vi "2020_day11.vi"() -> ()   [LabVIEW 2021]
uses:
  <userlib>/_OpenG.lib/array/array.llb/Search 1D Array (String)__ogtk.vi
panel:
  out "Task 1 (# od Occupied Seats)":i32
  out "Array 2":string[][](array[string])
  out "Array":string[][](array[string])
  in  "Switch":bool caption="Ex. Data  vs.  User Data"
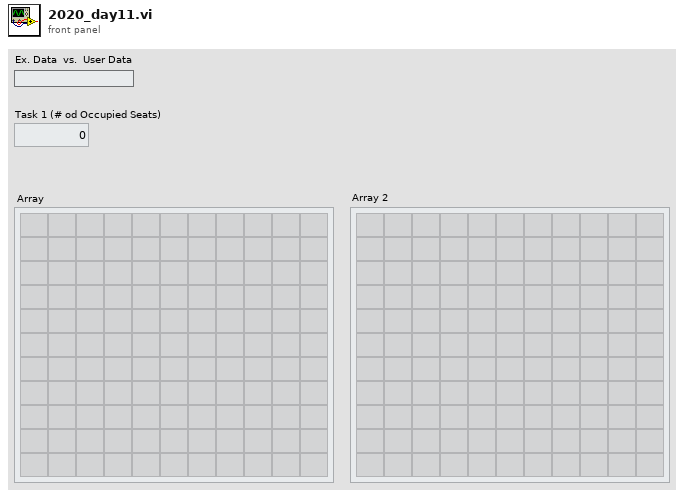
[diagram p1: front panel]
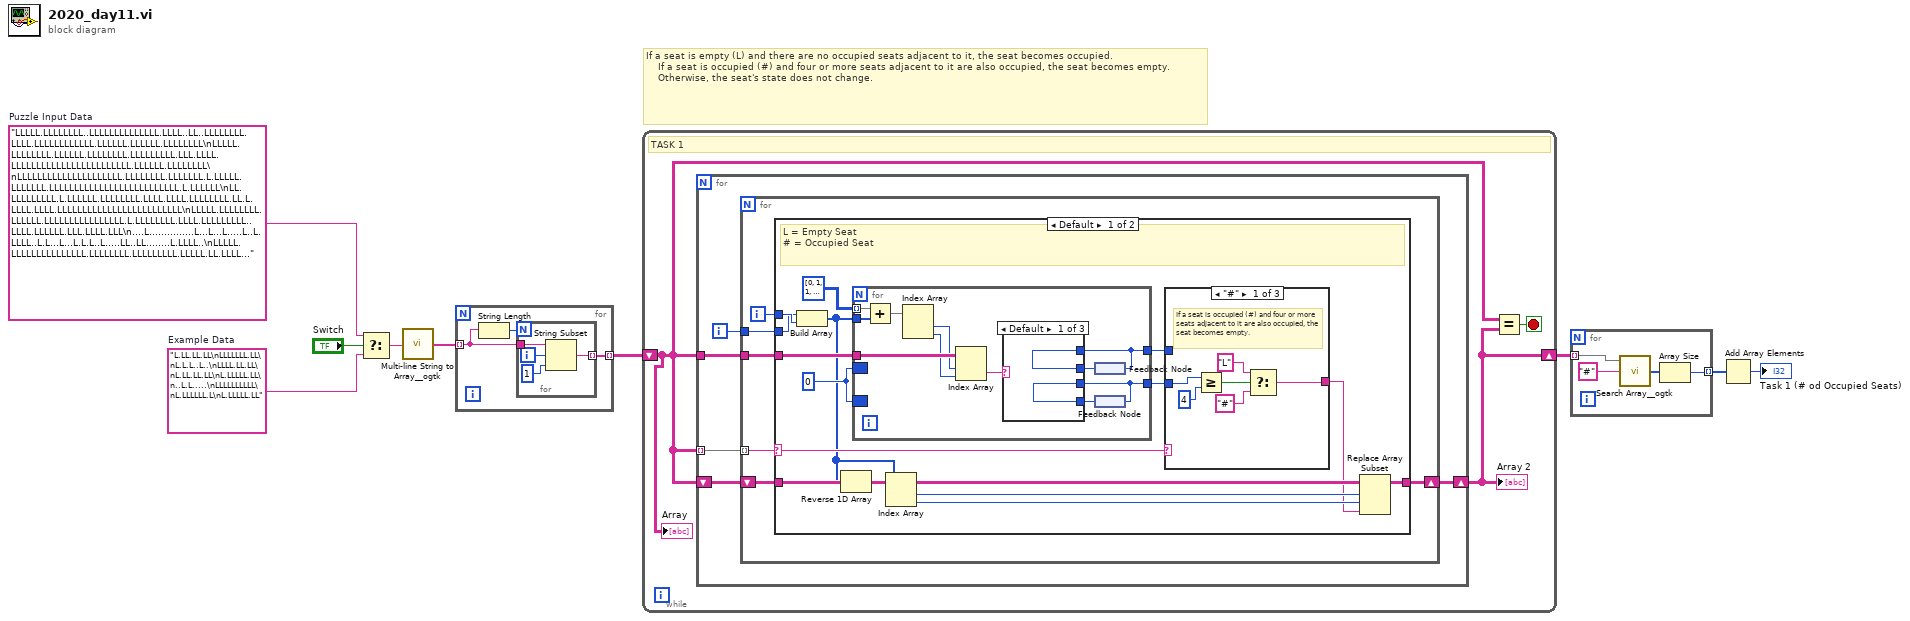
[diagram p0: block diagram]
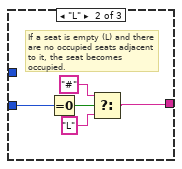
[diagram p2: hidden frame]
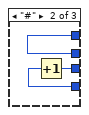
[diagram p4: hidden frame]
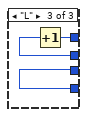
[diagram p5: hidden frame]
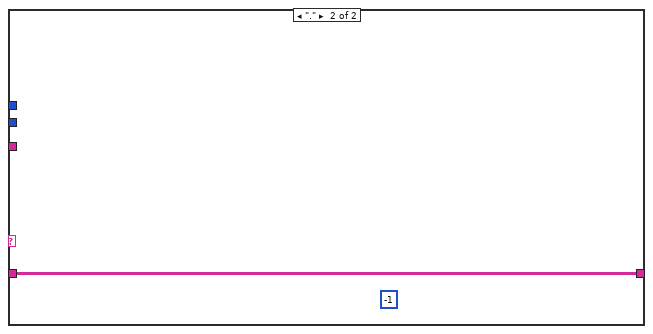
[diagram p6: hidden frame]
diagram:
  w7 = "LLLLL.LLLLLLLL..LLLLLLLLLLLLLL.LLLL..LL..LLLLLLLL.LLLL.LLLLLLLLLLLL.LLLLLL.LLLLLL.LLLLLLLL\nLLLLL.LLLLLLLL.LLLLLL.LLLLLLLL.LLLLLLLLL.LLL.LLLL.LLLLLLLLLLLLLLLLLLLLLLLL.LLLLLL.LLLLLLLL\nLLLLLLLLLLLLLLLLLLLLL.LLLLLLLL.LLLLLLL.L.LLLLL.LLLLLLL.LLLLLLLLLLLLLLLLLLLLLLLLLL.L.LLLLLL\nLL.LLLLLLLLL.L.LLLLLL.LLLLLLLL.LLLL.LLLL.LLLLLLLL.LL.L.LLLL.LLLL.LLLLLLLLLLLLLLLLLLLLLLLLL\nLLLLL.LLLLLLLL.LLLLLL.LLLLLLLLLLLLLLLL.L.LLLLLLLL.LLLL.LLLLLLLLL..LLLL.LLLLLL.LLL.LLLL.LLL\n....L...............L...L...L.....L..L.LLLL..L.L...L...L.L.L..L.....LL..LL........L.LLLL..\nLLLLL.LLLLLLLLLLLLLLL.LLLLLLLL.LLLLLLLLL.LLLLL.LL.LLLL.LLLL.LL.L.LLL.LLLLLLLLLLLL.LLLLLLLL\nLLLLLLLLLLLLLL.L.LLLL.LLLLLLLL.LLLLLLLLLLLLLLLLLL.L.LLLLLLLLLLLL.LLLLLLLLLLLLLLLLLLLLLLLLL\nLLLLL.LLLLLLLL.LLLLLLLLLLLLLLL.LLLL.LLLLLLLLLLL.LLLLLLLLLLLLLLLLLLLLLLLLLLLLLLLLL.LLLLLLLL\nLLLLLLLLLLLLLL.LLLLLL.LLL.LLLLLLLLL.L.LLLLLLLLLLL.LLLL.LLLLLLLLL.LLLLLLLLL..LLLLL.LLLLLLLL\nLLLLLLLLLLLLLL.LLLLLL.LLLLLLLL.LLLL.LLLL.LL.LLLLL.LLLL.LLLLLLLLL.LLLLLLLLL.LLLLLLLLLL.LLLL\nLLLLL.LLLLLLLLLLLLLLL.LLLLLLLL.LLLL.LLLL.LLLLLLLLLLLLL.LLLLLLLLL.LLLLLLLLLLLLLLLL.LLLLLLLL\nL..L..L.LLL...L.L.....L....L.LL..........L.L....LLL...L...L.LLL.L...L...L......L..L..L....\nLL.L.L..LLLL.LLLLLLLLLLLLLLLLL.LLLL..LLL.LLLLLLLL.LLLL.LLLLLLLLLL.LLLLLL.L.LLLLLLLLLLLLLLL\nLLLLLLLLLLLLLLLLLLLLLLLLLLLLLL.LLLL.LLL..LLLLLLLLLLLLLLLL.LLLLLL.LLL.LLL.L.LLLLLL.LLLLLLLL\nLLLLLLLLL.LLLLLLLLLLLLLL.LLLL..LLLLLLLLL.LLLLLLLL.LLLLLLLL.LLLLL.LLLLLLLLLLLLLLLLLLLLLLLLL\nLLLLL.LLLLLLLLLLLLLLL.LLLLLLLL.LL.LLLLLL.LLLLLLLL.LLLL.LLLLLLLLL.LLLLLLLLL.LLLLLL.LL.LLLLL\nLLL.L.LLLLLLLL.LLLLLL.LLLLLLLLLLLLL.LLLL.LLLLLLLL.LLLL.LL.LLLL.L.LLLL.LLL.LLLLLLL.LLLLLLLL\nLLLLL.LLLLLLLL.LLLLLL.LLLLLLLL.LLLL.LLLL.LLLLLLLLLLLLL.LLLLLLLLLLLLLLLLLLLLLLLLLL.LLLLLLLL\n.LLLL.LLLLLLLLLLLLLLL.LLLLLLLL.LLLL.LLLL.LLLLL.LLLLLLLLLLLLLLLLL.LLLLLLLLL.LLLLLL.LLLLLL.L\nLL....LL.L.L....L...........L........L...L.L.L.L.L.L.L...LLLL....L......L..LL.L...L...L..L\nLLLLL.LLLLLLLL.LLLLLL.L.LLLLLL.LLLLLLLLLLLLLLLLLLLL.LL.LLLLLLLLLLLLLLLLLLL.LLLLLL.LLLLLLLL\nLL.LL.LLLLLLLL.LLLLLL...LLLLLL.LLLL.LLLL.LLLLLLLL.LL.L.LLLLLLLLLLLLLLLLLLL.LLLLL..LLLLLLLL\nLLLLL.LLL.LLLL.LL.LLLLLLLLLLLL.LLLLLLLLL.LLLLLLLL.LLLL.LLLLLLLLLLLLLLLLLLL..LLL.LLL.LLLLLL\nLLLL.LLLLLLLLL.LLLLLL.LLLLLLLL.LLLLLLLLL.LLLLLLLLLLLLLLLLLLLLLLL.LLLLLLLLL.LLLL.L.LLLLLLLL\nLLLLLLLLLLLLLL.LLLLLL.LLLLLLLLLLLLL.LLLLLLLLLLLLL.LLLL.LLLLLLLLL.LLLLLLLLLLLLL.LL.L.LLLLLL\n.LLLLL..L.LL....L..LL.LLL.L.....LLL.LL..........L..L..LL..L..L.L..L.L.L..L.L...........L.L\nLLLLL.LLLLLLLL.LLLLLLLL.LLLLLL.LLLLLLLLL.LLLLLLLLLLLLL.LLLLLLLLL.LLLLLLLLL.LLLLLL.LLLL.LLL\nLLLLLLLLLLLLLLLLLLLLLLLLLLLLLL.LLL..LLLLLLLLLLLLLLLLLL.LLLLLL.LLLLLLLLLLLL.LLLLLLLL.LLLLLL\nLLL.L.LLLLLLLL.LLLLLLLLLLLLL.L.LLLL.LLLLLLLLLLLLL.LLLL.L.LLLLLLLLLLLLLLLLL.LL.LLL.LLLLLLLL\nLLLLLLLLLLLLLLLLLLLLL.LLLLLLLLLLLLL.LLLL.LLLLLLLL.LLLL..LLLLLLLL.LLLLLLLLL.LLLLLL.LLLLL.LL\nLLLLLLLLL.LLLL.LLLLLL.LLLLLLLL.LLLLLLLLLLLLLLLLLL.LLLL.L.LLLLLLL.LLLLLLLLLL.LLLLL.LLLLLLLL\nLLLLL.LLLLLLLLLLLLLLL.LLLLLLLLLLLLLLLLLL.LLLLLLLL.LLLL.LLLLLLLLLLLLL.LLLLL.LLLLLL.LLLL.LLL\nLLLLL.LLLLLLLL.LLLLLL.LLLLLLLLLLLLL.LLLL.LLLLLLLL.LLLL.LLLL.LLLLLLL.LLLLLL.LLLLLL.LLLLLLLL\nLLL.LLLLL....L..L..L....L.L..L....L..LL..L.........L......L..L....LL...L.L...LLLLL.....L.L\n.LLLL.LLLLLLLLLLLLLL.LLLLLLLLL.LLLLLLLLL.LLLLLLLL.LL.L.LLL.LLLLL.LLLLLLLLLLLLLLLLLLLLLLLLL\nLLL.LLLLLLLLL.LLLLLLLLLLLLLLLL.LLLL.LLLL.LLLLLLLL.LLLL.LLLLLLLLLLLLLLLLLLL.LLLLLL.LLLLLLLL\nLLLLLLLLLLLLLL.LLLLLL.LLLLLLLLLLLLLLLLL..LLLLLLLL.LLLL.LLLLLLL.L.LLLLLLLLL.LLLL.L.LLL.LLLL\nLLLLL.LLLLLLLL.LLLLLL.LLLLLLLLLLLLLLLLLLLLLLLLLLL.LLLL.LLLLLLL.L.LLLLLLLL.LLLLLLL..LLLLLLL\n....L...LL....L..L..L.L......LLL........L.LL..L.L...L...L..L....LLL..LL.LLL.LLL.L..L....L.\nLLLLLLLLLLLLLL.LLLLLL.LLLLLLL..LLLL.LLLL..LLLLLLLLLL.LLLLLLLLLLL..LLLLLL.LLLLLLLL.LLLLLLLL\nLLLLLLLLL.LLLLLLLLLLL.LLLLLLLLLLLLL.LLLL.LLLLLLLL.LLLL.LLLL.LLLL.LL.LLLL.L.LLL.LL.LLLL.LLL\nLLLLL.LL.LLLLL.LLLL.L.LLLLLLLL.LLLL.L.LLLLLLLLLLL.LLLL.LLLLLLLLL.LLLLLLLLL.LLLLLL.LLLLLLLL\nLLLLL.LLLLLLLLLLLLLLL.LLLLLLLL.LLL.LLLL..LLLLLLLL.LLLL.LLLLLLLLLLLLLLLLLLL.LLLLLL.LLLLLLLL\nL.LLL.LLLLLLLL.LL.LLLLLLLLLLLL.LLLL.LLLL.LL.L.LLL.LLLL.LLLLLLLL..LLLLLLLLL.LLLLLL.LLLLLLLL\n...LLLL..L...LLLL..LL...L.......L..LLL....L..........LL.L...LL.L.....L.....LL..L......LLLL\nL.LLL.LLLLLLLLLLLLLLL.LLLLLLLL.LLLLLL.LL.LLLLLLLLLLLLLLLLLLLL.LLLLL.LLLL.LLLLLLLL.LLLLLLLL\nLLLLL.LLLLLLLL.LLLLLL.LLLLLLLLLLLLL.LLLL..LLLLLLL.L.LL.LLLLLLL.LLLLLLLLLLL.LLLLLLLLLLLLLLL\nLLLLL.LLLLLLL..LLLLLLLLLLLLLLL.LLLLLLLLL.LLLLLLLL.LLLL.L.L...LLLLLLLLLLLLLLLLLLLLLLLLLLLLL\nLLLLLLL.LLLLL..LLLLLLLLLLLLLLLLLLLL.LLLL.LLLLLLLLLLLLLLLLLLLLLLL.LLLLLLLLLLLLLLLLLLLLLLLLL\n....LLL.L.......LL.....LL..L...LL.LLL......L..L..LL..LL.LL.L..L.LL.....L.L.L.L.....L..L...\nLLL.L.LLLLLLLL.LL.LLL.LLLLLLLL.LLLL.LLLLLLLLLLLLL.LLLLLLLL.LLLLL.LLLLLLLLLLLLLLLLLLLLLLLLL\nLLLLL.LLLLLLLL.LLLLLLLLLLLLLLL.LLLL.LLLLLLLLLLLLL.LLL..LLLLLLLLLLLLLLLLLLL.LLLLLL.LLLLLLLL\nLLLLL.LL.LLLLL.LLLLLL.LLLLLLLLLL.LL.LLLL.LLLLLLLLLLLLLLLLLLLLLLL.LLLLLLLLL.LLLLLL.LLLLLLLL\nLLLLL.LLLLLLLL.LLLLLL.LLLL.LLLLLLLLLLLLLLLLLLLLLL.LLLL.LLLLLLLLL.LLLLLLLLL.LLLLLL.LLLLLLLL\nLLLLL.LLLLLLLLLLLLLLL.LLLLLLLL.LLLLLLLLL.LLLLLLL..LLLL.LLLLLLL.LLLLLLLLLLLLLLLLLLLLLLLL.LL\nLLLLL.LLLLLLLL.LLL.LLLLLLLLLLL.LLLLLLLLLLLLLLLLLL.LLLL.LLLLLLLLL.LLLLLLLLL.LLLLLL.LLLLLLLL\nLLLLLLLLLLLLLL.LLLLLL.LL.LLLLL.LLLLLLLLL.LLLLLLLL.LLLL.LLLLLLLL..LLLLLLLL..LL.LLL.LLLLLLLL\nLLL..L.L.L..........LL....L...L.L.LLL.L.L..L.....L...L.LLL............L.L.L..L..........L.\nLLLLL.LLLLL..L.LLLLLL.LLLLLLLL.LLLL.LLLL.LLLLLLLLLLLLL.LLLLLLLLL.LL.LLLLLLLLLLLLLLLLLLLLLL\nL.LLL.LLLLLLLL.LLLLLL.LLLLLLLL.LLLLLLL.L.LLLLLLLLLLLLL.LLLLLLLLL.LLLLLLLLLLLLLL.L.LLLLLLLL\nLLLL..LLLLLLLLLLLLLLLLLLLLL.LL.LLLL.LLLL.LLLLLLLL.LLLLLLLLLLLLLLLL.LLLL.LL.LLLLLLLLLLLLLLL\nLLLL..LLLLLLLL.LLLLLL.LLLLLLLL.LLL.L.LLL.LLLLLLLLLLLLL.LLLLLLLLLLLLL.LLLLL.LLLLLL.LLLLLLLL\nLLLLLLLLLLLLLLLLLLLLL.LLLLLLLL.LLLLLLLLL.LLLLLLLL.LLLLLLLLLLLLLLLLLL.LLLLLLLLLLLL.LLLL.LLL\n.LLLL.LLL.LLLLLLLLLLL.LLLL.LLL..LLLLLLLL.LLLLLLLLLLLLL.LL.LLLLLLLLLLLLLLLLLLLLL.L.LLLLLLLL\nLL.LL.LLLLLLLL.LLLLLLLLLLLLLLL.LLLL.LLLLLLLLLLLLLLLLLL.LLLLLLLLL.LLLLLLLLLL.LLLLL.LL.LLLLL\nLLLLL.LLLLLLLL.LLL.LL..LLLLLLL.LLLL.LLLL.LLLLLLLL.LLLLLLLLLLLLLL.LLLLLLLLL.LLLLLLLL.LLLLLL\n...L.L.........L............L...LLL.L.L.L....L..LL.LL...........L.LL.L.....LL.L.L..L..L...\nLLLLL.LLLLLLLL.LLLLLL.LLLLLLLLLLLLL.LL.L.LLLLLLLL.LLLLLLLLL.L.LLLLLLLLLLLL.LLLLLL.LLLLLLLL\nLLLLLLLLLLLL..LLLLLLLLLL.LLLLL.LLLL.LLLL.LLLLLLLL.LLLL.LL.LLLLLLLLLLLLLLLL.LLLLLL.LLL.LLLL\nLLLLLLLLLLLLLL.LLLLLLLLLLLLLLL.L.LL.LLLL.LLLLLLLLLLLLLLLLLLLLLLL..LLLLLLLL.LLLLLLLLLLLLLLL\nLLLLL.LLLLLLLLLLLLLLL.LLLLLLLL.LLLL.LLLL.LL..LLLL.LLLLLLLLLLLLLL.LLLLLLLLL.LLLLLL.L.LLLL.L\nLLLLLLLLLL.LLL.LLLLLL.L.LLLLLL.LLLL.LLLL.LLL.LLLL.LLLLLLLLLLLLLL.LLLLLLLLL.LLLLLLLLLLLLLLL\nLLLLL.LLLLLLLL.LLLLLL.LLLLLLLL.LLLLLLLLLLLLLLLLLL.LLLL.LLLLLLLLL.LLLLLL.LL.LLLLLL.LLLLLLLL\nLLLLL.LLLL.LLL.LLLLLLLLLLLLLLL.LLLL.LLLL.LLLLLLLLLLLLL.LLLLLLLLL.L.LLLLLLL.LLLLLL.LLLLLLLL\nL.LLLLLLLLLLLL.LLLLLL.LLLLLL.L.LLLLLLLLL.LL.LLLLL.LLLL.LLLLL.LLLLLLL.LLLLLLLLLLLLL.LLLLLLL\n.......L.LL.LLL.L.L.....LL.LL.L....L...LL...L......L..L.L..L...L.....L.LL.L.L.LL.L.L......\nLLLLL.LLLLLLLL.LLLLLL.LLLLLLLL.LLLL.LLLLLLLLLLLLL.LLLL.LLLLLLLLL.LLLLLLLLL.LLLLLL.LLL.LLLL\nLLLLL.LLLLLLLLLLLLLLL.LLLLLLLL.LLLL.LLLLLLLLLLLLL.LLLL.LLL.LLLLL.L.LLLLLLL..LL.L.LLLLLLLLL\nLLLLL.L.LLLLLL.LLLLLLLLLLLL.LLLLLLL.LLLLLLLLLLLLL.LLLLLLLLLL.LLL.LLLLLLLLL.LLLLLLLLLLL.LLL\nLLLLLLLLLLLLLL.LLLLLL.LLLLLLLL.LLL...LLL.LL.LLLLL.LLLL.LLLLLLLLL..LLLLLLLL.LLLLLL.LLLLLLLL\nLLLLLLLLLLLLLL.LLLLLL.LLL.LLLLLLLLLLLLLL.LLLLLLLL.LLLL.LLLL..LLL.LLLLLLLLL.LLLLLL.LLLLLLLL\nLLLLL.LLLLLLLL.LLLLL..LLL..LLL.LLLLLLLLL.LLLLLLLL.LLLLLLLLLLLLLLLLLLLLLLLL.LLLLLL.LLLLLLLL\nLLLLL.LLLLLLLL.LLLLLL.LL.LLLLLLLLLLLLLLL.LLLLLLLL..LLLLLLLLLLLLL.LLLLLLLLLLLLLLLL.LLLLLLLL\n...LL.L..L............LL.LL.....L.L.L..LLLL.L....L.L...L..LL.....LL.LL.L.L..LL..L..LL.L.L.\nLLLLLLLLLLLLLL.LLLLLL.LLLLLLLL.LLLL.LLLL.L.LLLLLLLLLLLLLLLLLLLLL.LLLLLLLLLLLLLLLLLLLLLLLLL\nLLLLLLLLLLLLLLLLLLLLL.LLLLLLLLLLLLL.LL.L.LLLLLLLL.LLLL.LLLLLLLLLLLLLLLLLLL.LLLLLLLLLLLLLLL\nLLLLLLL.LL.LLL.LLLLLLLLLLLLLLL.LLLL..LLL.LLLLLLLLLLLLLLLLLLLLLLL..LLLLLLLLLLL.LLLLLLLLLLLL\nLLLLLLLLLLLLLLLLLLL.L.LLLLLLLL.LLLLLLLLLLLLLLL.LLLLLLL.LLLLLLLLL.LLLLLLLLL.LLLLLLLLLLLLLLL\nLLLLL..LLLLLLL.LLLLLL.LLLLLLLLLLLLL.LLLL.LLLLLLLLLLLLLLLLLLLLLLLLLLLL.LL.L..LLLLL.LLLLLLLL\nLLLLLLLLLLLLLLL.LLLLL.LLLLLLLL..LLL.LLLL.LLLLLLLLLLLLLLLLLLLLLLL.LLLLLLLLL.LLLLLLLLLLLLLLL\nLLL.L.LLLLLLLL.LLLLLLLLLLLLLLLLLLLLLLLLL.L.L.LLL.LLLLL.LLLLLLLLL.LLLLLLLLL.LLLLLL.LLLLLLLL\nLLLLL.LLLLLLLL.LLLLLLLLLLLLLLL.LLLL.LLLL.LLLLLLLLLLLLL...LLLLLLL.LLLLLLLLL.LLLLLL.LLLLLLLL\n.LLLL.LLLLLLLLLLLLLL..LLLLLLL.LLLLL.LLLL.LLLLLLLLLL.LL.LLLLLLLLLLLLLLLLLLL.LLLL...LLLLLLLL\nLLLLLLLLLLLLLLLLLLLL..LLLLLLLL.LLLLLLLLL.LLLLLLLLLLLLLLLLLLLLLLL.LLLLLLLLL..LLLLL..LLLLLLL\nLLLLLLLLLLLLLL.LLLLLL.LLLLLLLLLLLLLLLLLL.LLLLL.LL.LL.L.LLLLLLLLL.LLLLLLLLL.LLLLLLLLLLLLLLL\nLL.LL.LLLLLLLL.LLLLLL.LLLLLLLL.LLLL.L.LL.LLLLLLLL.LLLL.LLLLLLL...LLLLLLLLL.LLLLLL.LL.LLLLL\nLLLLL.LLLLLLLL.LLLLLL.LLLLL.LLLLLLL.LLLLLLLL.LLLLLLLLL.LLLLLLLLL.LLLLLL..L.LLLLLL.LLLLLLLL\nLLLLL.LLLLLLLL.LLLLLLLLLL.LLLLLLLLL.LLLL.LLLLLLLL.LLL..LLLLLLLLL.LLLLLLLLL.LLLLLL.LLLLLLLL"  # Puzzle Input Data
  w8 = "L.LL.LL.LL\nLLLLLLL.LL\nL.L.L..L..\nLLLL.LL.LL\nL.LL.LL.LL\nL.LLLLL.LL\n..L.L.....\nLLLLLLLLLL\nL.LLLLLL.L\nL.LLLLL.LL"  # Example Data
  # "If a seat is empty (L) and there are no occupied seats adjacent to it, the seat becomes occupied.\n    If a seat is occupied (#) and four or more seats adjacent to it are also occupied, the seat becomes empty.\n    Otherwise, the seat's state does not change."
  n1 = Select(t=w7, s="Switch", f=w8) -> (s? t:f=w6:string)
  n2 = call <userlib>:"Multi-line String to Array__ogtk.vi"("string"=w6) -> ("lines"=w5:string[])
  n3 = for {
    tunnel: w5 -> [w11] mode=indexing
    tunnel: [w10] -> w4 mode=indexing
    n4 = String Length(string=w11) -> (length=w12:i32)
    n5 = for {
      N: w12 -> [_]
      tunnel: w11 -> [w16]
      tunnel: [w14] -> w10 mode=indexing
      i -> [w15]
      n6 = String Subset(string=w16, offset (0)=w15, length (rest)=1 ("length (rest)")) -> (substring=w14:string)
    }
  }
  n7 = while {
    shift-right: [w18] -> w3
    shift-left: w4 -> [w17]
    stop <- w19 stop-if-true
    # "TASK 1"
    n8 = for {
      tunnel: w17 -> [w24] mode=indexing
      tunnel: w17 -> [w22]
      shift-right: [w20] -> w18
      shift-left: w17 -> [w21]
      i -> [w23]
      n9 = for {
        tunnel: w24 -> [w30] mode=indexing
        tunnel: w23 -> [w25]
        tunnel: w22 -> [w27]
        shift-right: [w28] -> w20
        shift-left: w21 -> [w29]
        i -> [w26]
        n10 = case shown="Default" w30 {
          selector: w30 -> [w39 _]
          tunnel: w29 -> [w36 w76]
          tunnel: [w34 w76] -> w28
          tunnel: w27 -> [w41 _]
          tunnel: w26 -> [w44 _]
          tunnel: w25 -> [w43 _]
          frame Default {
            w40 = 0
            # "L = Empty Seat\n# = Occupied Seat"
            n11 = Build Array(w43, w44) -> (w31:i32[])
            n12 = Reverse 1D Array(array=w31) -> ()  [unwired: 1 out]
            n13 = for {
              tunnel: i32[][] [[0, 1], [1, 0], [0, -1], [-1, 0], [-1, 1], [-1, -1], [1, -1], [1, 1]] -> [w67] mode=indexing
              tunnel: w31 -> [w66]
              tunnel: w41 -> [w64]
              tunnel: [w59] -> w38
              border: w40 -> [_]
              border: w40 -> [_]
              tunnel: [w57] -> w32
              n14 = Add(x=w67, y=w66) -> (x+y=w65:i32[])
              n15 = Index Array(array=w65) -> (element #1=w63:i32, element #2=w62:i32)  [unwired: 2 in]
              n16 = Index Array(array=w64, index (row)=w63, index (col)=w62) -> (element=w61:string)
              n17 = feedback #1() -> (w60:i32)
              n18 = feedback #2() -> (w58:i32)
              n19 = case shown="Default" w61 {
                tunnel: [w69 w72 w75] -> w59
                tunnel: w60 -> [w69 w72 w74]
                tunnel: [w68 w70 w73] -> w57
                tunnel: w58 -> [w68 w71 w73]
                frame Default {
                }
                frame "#" {
                  n20 = Increment(x=w71) -> (x+1=w70:i32)
                }
                frame "L" {
                  n21 = Increment(x=w74) -> (x+1=w75:i32)
                }
              }
              n22 = feedback-in #1(w59) -> ()
              n23 = feedback-in #2(w57) -> ()
            }
            n24 = Index Array(array=w31) -> (element #1=w37:i32, element #2=w35:i32)  [unwired: 2 in]
            n25 = case shown="\"#\"" w39 {
              selector: w39 -> [_ _ w56]
              tunnel: w38 -> [_ _ _]
              tunnel: w32 -> [w47 w55 _]
              tunnel: [w48 w51 w56] -> w33
              frame "#" {
                # "If a seat is occupied (#) and four or more seats adjacent to it are also occupied, the seat becomes empty."
                n26 = Greater Or Equal?(x=w47, y=4 ("x")) -> (x >= y?=w45:bool)
                n27 = Select(t="L", s=w45, f="#") -> (s? t:f=w48:string)
              }
              frame "L" {
                # "If a seat is empty (L) and there are no occupied seats adjacent to it, the seat becomes occupied."
                n28 = Equal To 0?(x=w55) -> (x = 0?=w54:bool)
                n29 = Select(t="#", s=w54, f="L") -> (s? t:f=w51:string)
              }
              frame ".", Default {
              }
            }
            n30 = Replace Array Subset(array=w36, new element=w33, index (row)=w37, index (col)=w35) -> (w34:string[][])
          }
          frame "." {
            (unwired) -1
          }
        }
      }
    }
    "Array 2" <- w18
    n31 = Equal?(x=w17, y=w18) -> (x = y?=w19:bool)
    "Array" <- w17
  }
  n32 = for {
    tunnel: w3 -> [w79] mode=indexing
    tunnel: [w77] -> w2 mode=indexing
    n33 = call-poly <userlib>:"Search Array__ogtk.vi"("Array"=w79, "Element Data"="#") -> ("Indices of Elements"=w78:i32[])  [unwired: 7 in]
    n34 = Array Size(array=w78) -> (size(s)=w77:i32)
  }
  n35 = Add Array Elements(numeric array=w2) -> (sum=→"Task 1 (# od Occupied Seats)":i32)
